vi "NicmosCloseSynchronization.vi"(2 "Synchronization":T1, 9 "error out":errorcluster caption="error in (no error)") -> (6 "error in (no error)":errorcluster caption="error out")   [LabVIEW 2009]
uses:
  Controls/NicmosSynchronization.ctl
  Controls/NICMOS.COMMAND.ctl
  Controls/NICMOS.COMMANDBASIC.ctl
  Controls/NICMOS.READOUT.ctl
  Controls/NICMOS.FILTERCOMMAND.ctl
  Controls/NICMOS.FILTER.ctl
  Controls/NICMOS.STATE.ctl
  Controls/NICMOS.DATA.ctl
  Controls/NICMOS.RAW.ctl
  Controls/NICMOS.TEMPERATURE.ctl
  Controls/NICMOS.MASKBANKS.ctl
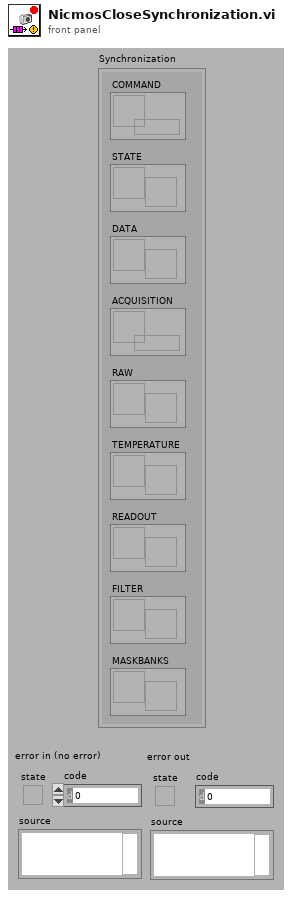
[diagram p1: front panel]
types:
  T1 = typedef "NicmosSynchronization.ctl" = cluster{"COMMAND":refnum<queue>, "STATE":refnum<notifier>, "DATA":refnum<notifier>, "ACQUISITION":refnum<queue>, "RAW":refnum<notifier>, "TEMPERATURE":refnum<notifier>, "READOUT":refnum<notifier>, "FILTER":refnum<notifier>, "MASKBANKS":refnum<notifier>}
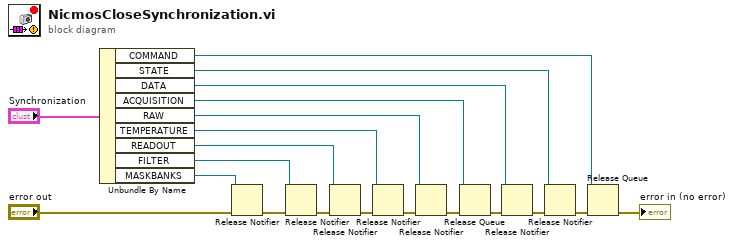
[diagram p0: block diagram]
diagram:
  n1 = Unbundle By Name("Synchronization") -> ("COMMAND"=w14:refnum<queue>, "STATE"=w15:refnum<notifier>, "DATA"=w16:refnum<notifier>, "ACQUISITION"=w4:refnum<queue>, "RAW"=w17:refnum<notifier>, "TEMPERATURE"=w18:refnum<notifier>, "READOUT"=w19:refnum<notifier>, "FILTER"=w7:refnum<notifier>, "MASKBANKS"=w1:refnum<notifier>)
  n2 = Release Notifier(notifier=w1, error in (no error)="error out") -> (error out=w2:errorcluster)  [unwired: 1 in, 2 out]
  n3 = Release Notifier(notifier=w7, error in (no error)=w2) -> (error out=w8:errorcluster)  [unwired: 1 in, 2 out]
  n4 = Release Notifier(notifier=w19, error in (no error)=w8) -> (error out=w12:errorcluster)  [unwired: 1 in, 2 out]
  n5 = Release Notifier(notifier=w18, error in (no error)=w12) -> (error out=w11:errorcluster)  [unwired: 1 in, 2 out]
  n6 = Release Notifier(notifier=w17, error in (no error)=w11) -> (error out=w6:errorcluster)  [unwired: 1 in, 2 out]
  n7 = Release Queue(queue=w4, error in (no error)=w6) -> (error out=w5:errorcluster)  [unwired: 1 in, 2 out]
  n8 = Release Notifier(notifier=w16, error in (no error)=w5) -> (error out=w10:errorcluster)  [unwired: 1 in, 2 out]
  n9 = Release Notifier(notifier=w15, error in (no error)=w10) -> (error out=w9:errorcluster)  [unwired: 1 in, 2 out]
  n10 = Release Queue(queue=w14, error in (no error)=w9) -> (error out=→"error in (no error)":errorcluster)  [unwired: 1 in, 2 out]
